vi "CMWsubscribeBOOL(noinit).vi"(8 "error in":errorcluster, 9 "Timeout?":bool, 10 "Data":variant, 11 "CMWboolIN":refnum<class "CMWSubscribe.lvclass">) -> (0 "error out":errorcluster, 2 "CMWbool":string, 3 "CMWboolOUT":refnum<class "CMWSubscribe.lvclass">)   [LabVIEW 2014]
uses:
  <userlib>/_RADE/RIO/CMW/classes/CMWSubscribe/CMWSubscribe.lvclass
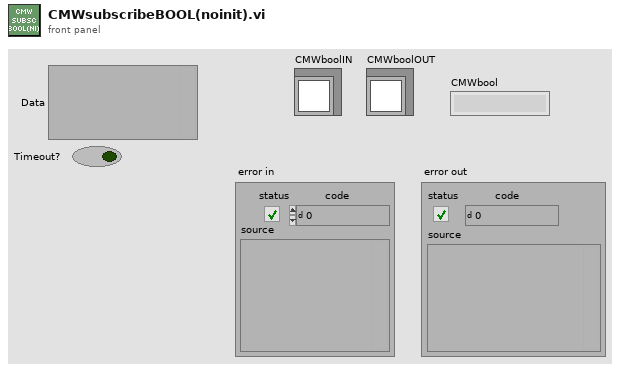
[diagram p1: front panel]
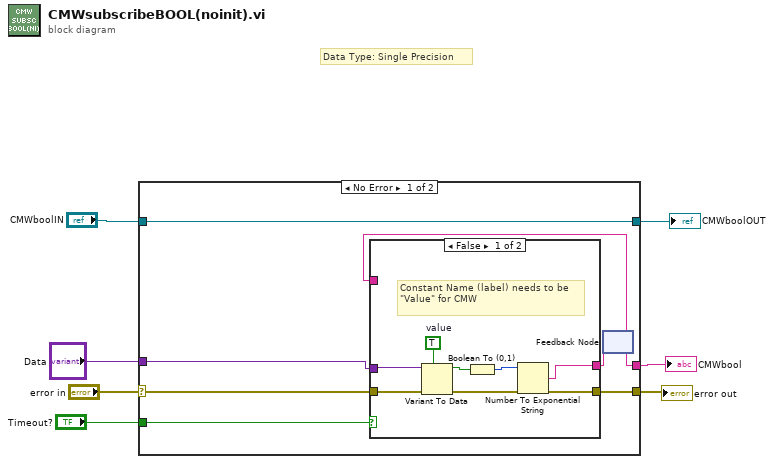
[diagram p0: block diagram]
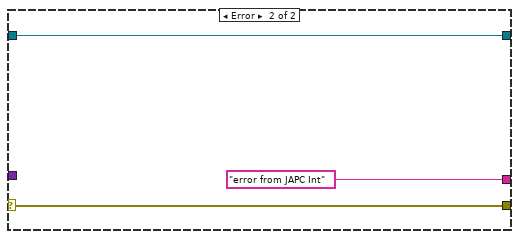
[diagram p3: hidden frame]
diagram:
  # "Data Type: Single Precision"
  n1 = case shown="No Error" "error in" {
    selector: "error in" -> [w10 w26]
    tunnel: [w14 w26] -> w5
    tunnel: "CMWboolIN" -> [w11 w25]
    tunnel: [w11 w25] -> w4
    tunnel: [w12 "error from JAPC Int"] -> w3
    tunnel: "Data" -> [w9 _]
    tunnel: "Timeout?" -> [w8 _]
    frame No Error {
      n2 = feedback #1() -> (w12:string)  [unwired: 1 in]
      n3 = case shown="False" w8 {
        tunnel: w10 -> [w21 w23]
        tunnel: [w19 w23] -> w14
        tunnel: w9 -> [w20 _]
        tunnel: [w18 w22] -> w13
        tunnel: w12 -> [_ w22]
        frame False {
          w17 = TRUE  # value
          # "Constant Name (label) needs to be \"Value\" for CMW"
          n4 = Variant To Data(error in=w21, type=w17, Variant=w20) -> (data=w16:bool, error out=w19:errorcluster)
          n5 = Boolean To (0,1)(Boolean=w16) -> (0, 1=w15:i16)
          n6 = Number To Exponential String(number=w15) -> (E-format string=w18:string)  [unwired: 3 in]
        }
        frame True {
          # "Subscription Timed Out"
        }
      }
      n7 = feedback-in #1(w13) -> ()
    }
    frame Error {
    }
  }
  "error out" <- w5
  "CMWboolOUT" <- w4
  "CMWbool" <- w3
